vi "Vision Processing.vi"(4 "error in (no error)":errorcluster) -> ()   [LabVIEW 2013]
doc: "This VI runs in parallel to other tasks. It gets images from the camera, processes them for color or shape and use that information to affect robot behavior."
uses:
  Robot Global Data.vi
  Example_Code/2014 Target Detection/TargetType.ctl
panel:
  in  "Score cutoff":dbl=50.0
  out "Loop time (ms)":u32
  out "Distance (ft)":dbl
  out "Scores.State":T1
  in  "Color Components":T2={"Hue"={100.0, 201.0}, "Sat"={0.0, 255.0}, "Val"={234.0, 255.0}} {"Val" scale=0.0..255.0; "Sat" scale=0.0..255.0; "Hue" scale=0.0..255.0 scale format="%#_3g"}
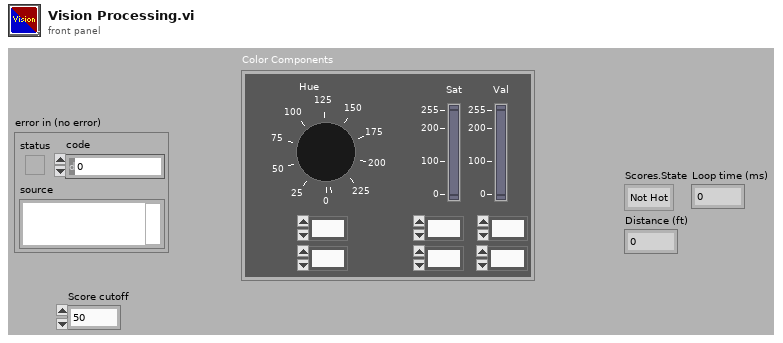
[diagram p1: front panel]
types:
  T1 = typedef "TargetType.ctl" = enum16{"Not Hot", "Hot"}
  T2 = cluster{"Hue":cluster{dbl, dbl}, "Sat":cluster{dbl, dbl}, "Val":cluster{dbl, dbl}}
  T3 = typedef "Image Type" = u32
  T4 = typedef "WPI_CameraDevRef.ctl" = cluster{"Camera Address":string, "CameraStatus":errorcluster, "Acquire Image Notifier":refnum<notifier>}
  T5 = typedef "IMAQ Image.ctl" = refnum<image>
  T6 = typedef "WPI_CameraImageSize.ctl" = enum16{"640x480", "320x240", "160x120"}
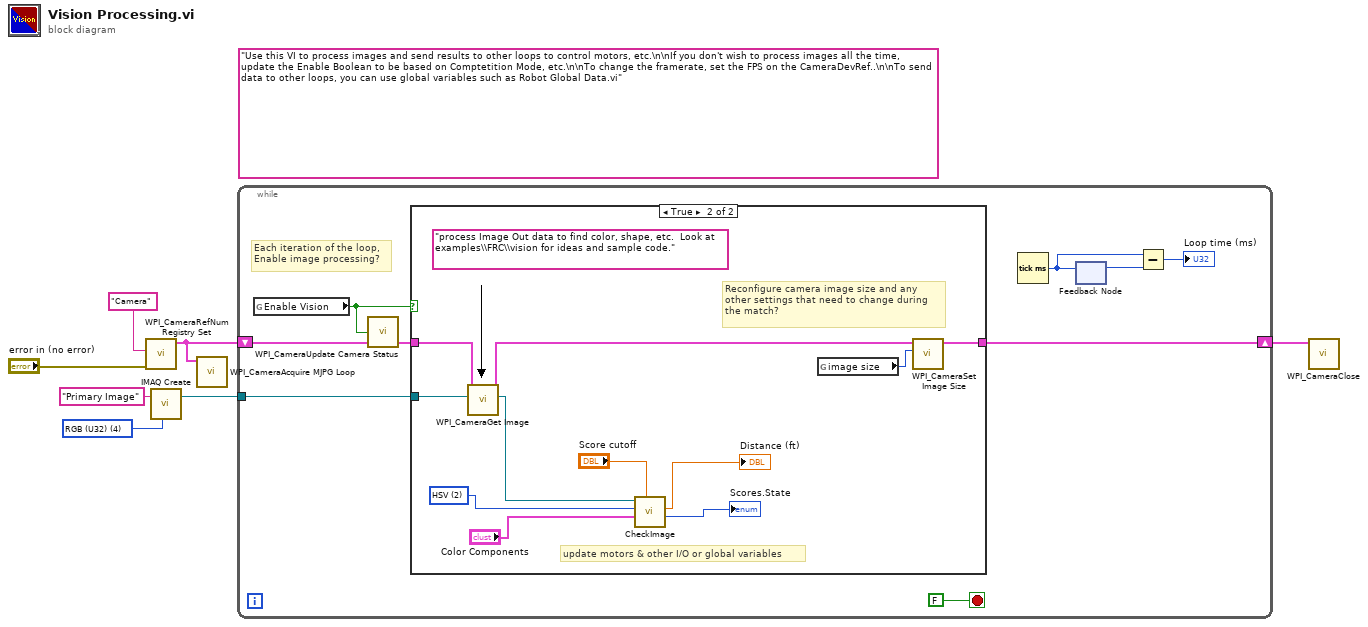
[diagram p0: block diagram]
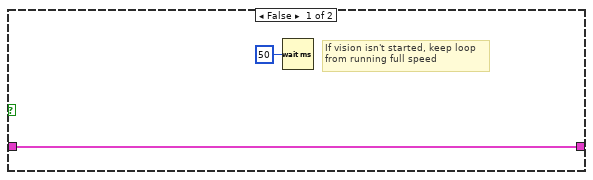
[diagram p2: hidden frame]
diagram:
  (unwired) "Use this VI to process images and send results to other loops to control motors, etc.\n\nIf you don't wish to process images all the time, update the Enable Boolean to be based on Comptetition Mode, etc.\n\nTo change the framerate, set the FPS on the CameraDevRef..\n\nTo send data to other loops, you can use global variables such as Robot Global Data.vi"
  w7 = T3 4 items=["Grayscale (U8)", "Grayscale (I16)", "Grayscale (SGL)", "Complex (CSG)", "RGB (U32)", "HSL (U32)", "RGB (U64)"] ("Image Type")
  n1 = call <vilib>:"WPI_CameraRefNum Registry Set.vi"("error in (no error)"="error in (no error)", "refnum name"="Camera") -> ("CameraDevRef"=w3:T4)  [unwired: 1 in, 8 out]
  n2 = call "IMAQ Create"("Image Name"="Primary Image", "Image Type"=w7) -> ("New Image"=w5:T5)  [unwired: 2 in, 2 out]
  n3 = call <vilib>:"WPI_CameraAcquire MJPG Loop.vi"("CameraDevRef"=w3) -> ()  [unwired: 11 in]
  n4 = while {
    shift-right: [w15] -> w2
    shift-left: w3 -> [w13]
    tunnel: w5 -> [w14]
    stop <- FALSE stop-if-true
    # "Each iteration of the loop,\nEnable image processing?"
    n5 = global read "Robot Global Data.vi" "Enable Vision"() -> (w11:bool)
    n6 = call <vilib>:"WPI_CameraUpdate Camera Status.vi"("CameraDevRef In"=w13, "Enable Vision"=w11) -> ("CameraDevRef Out"=w12:T4)  [unwired: 3 in]
    n7 = case shown="True" w11 {
      tunnel: w14 -> [_ w28]
      tunnel: [w18 w29] -> w15
      tunnel: w12 -> [w18 w26]
      frame False {
        # "If vision isn't started, keep loop\nfrom running full speed"
        n8 = Wait (ms)(milliseconds to wait=u32 50) -> ()  [unwired: 1 out]
      }
      frame True {
        w21 = u16 2 items=["RGB", "HSL", "HSV", "HSI"] ("Color System")
        (unwired) "process Image Out data to find color, shape, etc.  Look at examples\\FRC\\vision for ideas and sample code."
        # "update motors & other I/O or global variables"
        # "Reconfigure camera image size and any\nother settings that need to change during\nthe match?"
        n9 = call <vilib>:"WPI_CameraGet Image.vi"("Image"=w28, "CameraDevRef"=w26) -> ("Image Out"=w23:T5, "CameraDevRef Out"=w25:T4)  [unwired: 1 in, 7 out]
        n10 = call "CheckImage.vi"("Score cutoff"="Score cutoff", "Color Components"="Color Components", "Color System"=w21, "Image"=w23) -> ("Scores.State"=→"Scores.State":T1, "Distance (ft)"=→"Distance (ft)":dbl)  [unwired: 4 in, 2 out]
        n11 = global read "Robot Global Data.vi" "image size"() -> (w27:T6)
        n12 = call <vilib>:"WPI_CameraSet Image Size.vi"("Image Size"=w27, "CameraDevRef"=w25) -> ("CameraDevRef Out"=w29:T4)  [unwired: 1 in, 8 out]
      }
    }
    n13 = Tick Count (ms)() -> (millisecond timer value=w9:u32)
    n14 = feedback-in #1(w9) -> ()
    n15 = feedback #1() -> (w10:u32)  [unwired: 1 in]
    n16 = Subtract(x=w9, y=w10) -> (x-y=→"Loop time (ms)":u32)
  }
  n17 = call <vilib>:"WPI_CameraClose.vi"("CameraDevRef"=w2) -> ()  [unwired: 1 in, 10 out]
